vi "Ventus - Query Error.vi"(8 "error in (no error)":errorcluster, 11 "VISA Refnum in":refnum<visa-resource-name>) -> (0 "error out":errorcluster, 2 "Error Status":string, 3 "VISA Refnum out":refnum<visa-resource-name>)   [LabVIEW 2020]
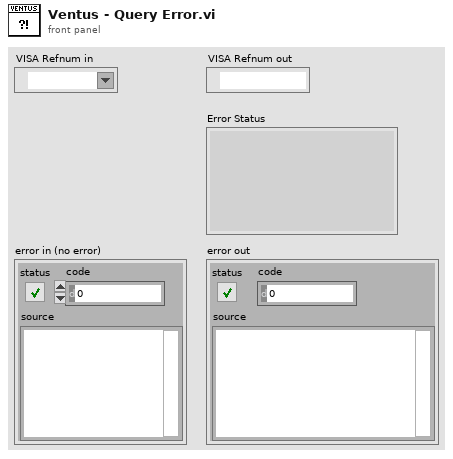
[diagram p1: front panel]
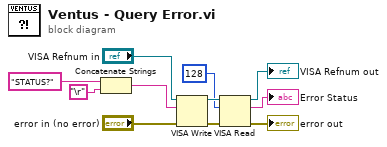
[diagram p0: block diagram]
diagram:
  n1 = Concatenate Strings("STATUS?", "\r") -> (w7:string)
  n2 = VISA Write(VISA resource name="VISA Refnum in", write buffer=w7, error in (no error)="error in (no error)") -> (VISA resource name out=w2:refnum<visa-resource-name>, error out=w3:errorcluster)  [unwired: 1 out]
  n3 = VISA Read(VISA resource name=w2, byte count=u32 128, error in (no error)=w3) -> (VISA resource name out=→"VISA Refnum out":refnum<visa-resource-name>, read buffer=→"Error Status":string, error out=→"error out":errorcluster)  [unwired: 1 out]
